vi "Variable@GetPointElement__Parameter.vi"(1 "ParamterIn":string) -> (0 "ParamterOut":string)   [LabVIEW 2020]
panel:
  in  "Axis":string(combo)
  in  "Point":string(combo)
  in  "Section":string(combo)
  in  "Variable":string(combo)
  in  "Confirm":bool
  # "Variable@GetPointElement $Variable=AXIS($Point)(,Section)\nAXIS is X,Y,Z,U,V,W,H,Delay,IO"
  # "Variable=X(Point)(,Section)\nVariable=Y(Point)(,Section)\nVariable=Z(Point)(,Section)\nVariable=U(Point)(,Section)\nVariable=V(Point)(,Section)\nVariable=W(Point)(,Section)\nVariable=H(Point)(,Section)"
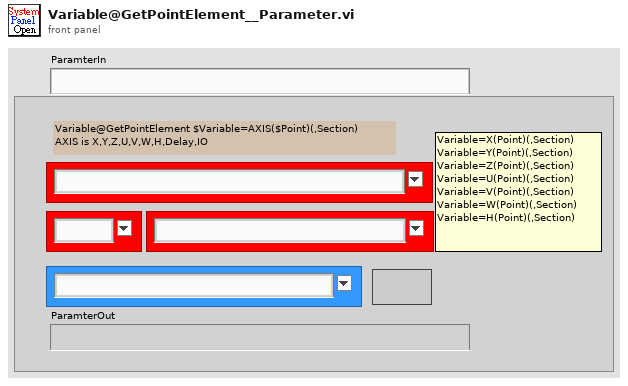
[diagram p1: front panel]
types:
  T1 = enum16{"Get", "UpdatePointS", "Init", "UpdateIndex", "GetCurrent&Index+1", "GetWithIndex", "ChkLast", "GetCurrent"}
  T2 = enum16{"Get", "Init", "Set", "Delete", "GetElement", "Inc", "Dec"}
  T3 = enum16{"Get", "Init", "Set", "Delete", "GetElement", "Inc", "Dec", "ReName"}
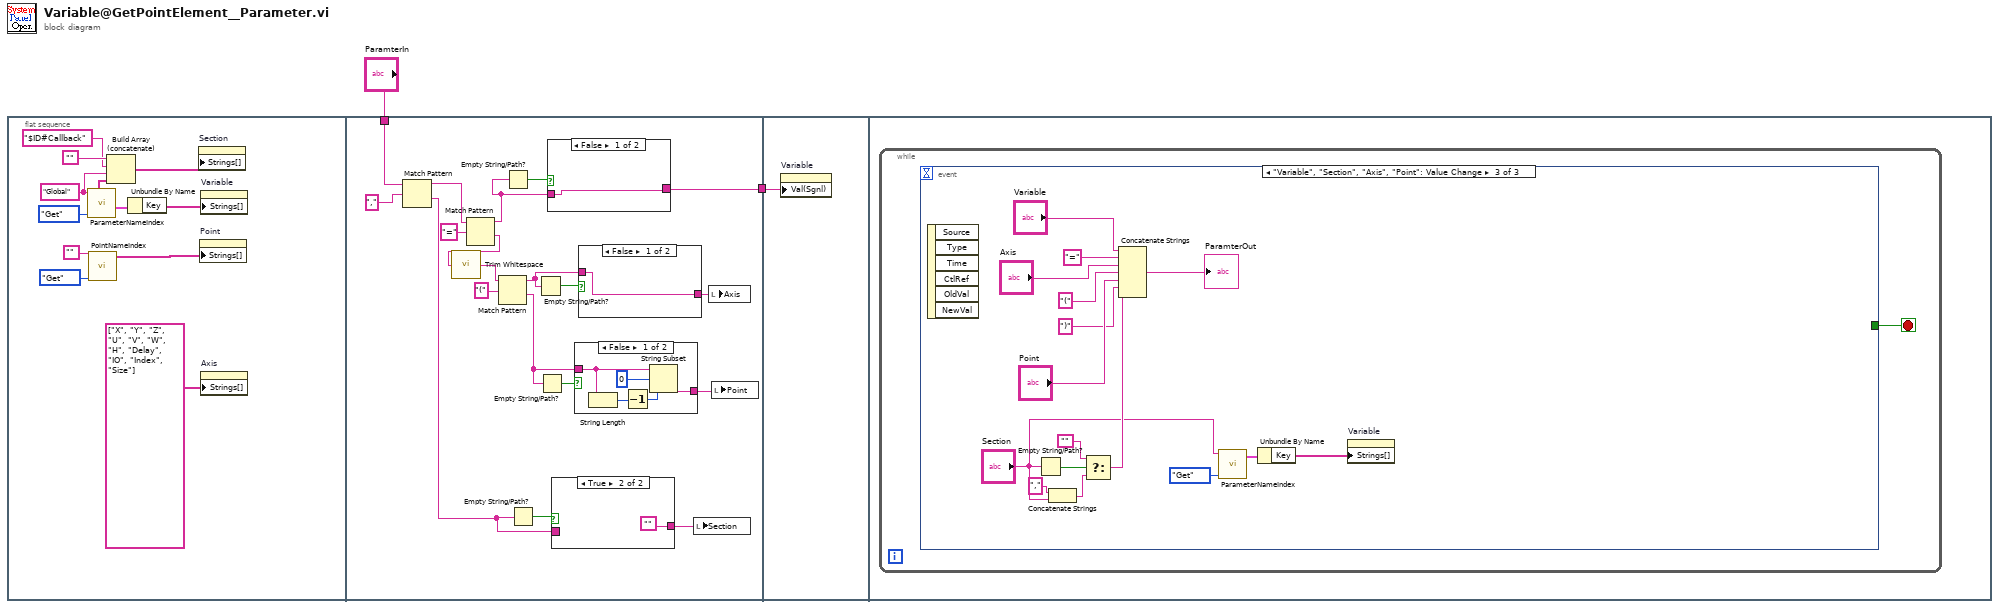
[diagram p0: block diagram]
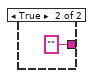
[diagram p2: hidden frame]
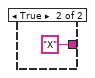
[diagram p3: hidden frame]
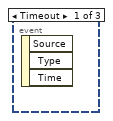
[diagram p6: hidden frame]
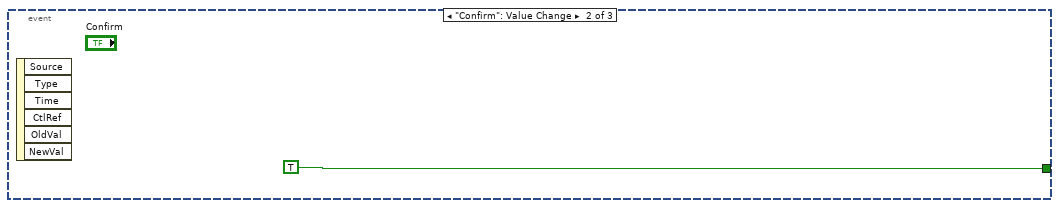
[diagram p7: hidden frame]
diagram:
  n1 = flat-sequence {
    tunnel: "ParamterIn" -> [w32]
    tunnel: [w28] -> w1
    tunnel: w1 -> [w46]
    frame #0 {
      w5 = "Global" ("VariableSection")
      n2 = call "ParameterNameIndex.vi"("OP"=T2."Get", "VariableSection"=w5) -> ("GlobalKeyValue"=w13:cluster{"Key":string[], "Value":string[]}, "SectionList"=w6:string[])  [unwired: 3 in, 5 out]
      n3 = call "PointNameIndex.vi"("OP"=T1."Get", "PointName"="") -> ("PointNameList"=w9:string[])  [unwired: 4 in, 5 out]
      n4 = Build Array (concatenate)("", "$ID#Callback" ("VariableSection"), w5, w6) -> (w4:string[])
      n5 = Unbundle By Name(w13) -> ("Key"=w12:string[])
      n6 = property on="Section" class="CmbBox"("Strings[]"=w4) -> ()  [unwired: 2 in, 2 out]
      n7 = property on="Point" class="CmbBox"("Strings[]"=w9) -> ()  [unwired: 2 in, 2 out]
      n8 = property on="Variable" class="CmbBox"("Strings[]"=w12) -> ()  [unwired: 2 in, 2 out]
      n9 = property on="Axis" class="CmbBox"("Strings[]"=string[] ["X", "Y", "Z", "U", "V", "W", "H", "Delay", "IO", "Index", "Size"] ("Strings []")) -> ()  [unwired: 2 in, 2 out]
    }
    frame #1 {
      n10 = Match Pattern(string=w32, regular expression=",") -> (before substring=w26:string, after substring=w29:string)  [unwired: 1 in, 2 out]
      n11 = Match Pattern(string=w26, regular expression="=") -> (before substring=w23:string, after substring=w20:string)  [unwired: 1 in, 2 out]
      n12 = call <vilib>:"Trim Whitespace.vi"("string"=w20) -> ("trimmed string"=w19:string)  [unwired: 1 in]
      n13 = Match Pattern(string=w19, regular expression="(") -> (before substring=w15:string, after substring=w17:string)  [unwired: 1 in, 2 out]
      n14 = Empty String/Path?(string/path=w23) -> (empty?=w33:bool)
      n15 = Empty String/Path?(string/path=w29) -> (empty?=w30:bool)
      n16 = Empty String/Path?(string/path=w15) -> (empty?=w22:bool)
      n17 = Empty String/Path?(string/path=w17) -> (empty?=w18:bool)
      n18 = case shown="False" w33 {
        tunnel: w23 -> [w44 w45]
        tunnel: [w44 w45] -> w28
        frame False {
        }
        frame True {
        }
      }
      n19 = case shown="True" w30 {
        tunnel: w29 -> [w42 _]
        tunnel: [w42 ""] -> w27
        frame False {
        }
        frame True {
        }
      }
      n20 = case shown="False" w18 {
        tunnel: [w38 "" ("ParamterIn")] -> w16
        tunnel: w17 -> [w36 _]
        frame False {
          n21 = String Length(string=w36) -> (length=w35:i32)
          n22 = Decrement(x=w35) -> (x-1=w34:i32)
          n23 = String Subset(string=w36, offset (0)=0, length (rest)=w34) -> (substring=w38:string)
        }
        frame True {
        }
      }
      n24 = case shown="False" w22 {
        tunnel: [w40 "X" ("ParamterIn")] -> w21
        tunnel: w15 -> [w40 _]
        frame False {
        }
        frame True {
        }
      }
      n25 = local write "Section"(w27) -> ()
      n26 = local write "Axis"(w21) -> ()
      n27 = local write "Point"(w16) -> ()
    }
    frame #2 {
      n28 = property on="Variable" class="CmbBox"("Val(Sgnl)"=w46) -> ()  [unwired: 2 in, 2 out]
    }
    frame #3 {
      n29 = while {
        stop <- w47 stop-if-true
        n30 = event shown="[2] \"Variable\", \"Section\", \"Axis\", \"Point\": Value Change" {
          selector: _ -> [_ _ _]
          dyn-events: _ -> [_ _ _]
          timeout: _ -> [_ _ _]
          tunnel: [_ TRUE _] -> w47
          event Timeout {
            n31 = event-data() -> ()  [unwired: 1 in, 3 out]
          }
          event "Confirm": Value Change {
            n32 = event-data() -> ()  [unwired: 1 in, 6 out]
          }
          event "Variable", "Section", "Axis", "Point": Value Change {
            n33 = event-data() -> ()  [unwired: 1 in, 6 out]
            n34 = Empty String/Path?(string/path="Section") -> (empty?=w62:bool)
            n35 = Concatenate Strings("," ("string"), "Section") -> (w60:string)
            n36 = Select(t="", s=w62, f=w60) -> (s? t:f=w54:string)
            n37 = Concatenate Strings("Variable", "=" ("string"), "Axis", "(" ("string"), "Point", ")" ("string"), w54) -> (→"ParamterOut":string)
            n38 = call "ParameterNameIndex.vi"("OP"=T3."Get", "VariableSection"="Section") -> ("SectionKeyValue"=w50:cluster{"Key":string[], "Value":string[]})  [unwired: 3 in, 6 out]
            n39 = Unbundle By Name(w50) -> ("Key"=w52:string[])
            n40 = property on="Variable" class="CmbBox"("Strings[]"=w52) -> ()  [unwired: 2 in, 2 out]
          }
        }
      }
    }
  }
